vi "Debug Transceiver.vi"(11 "UDPlog Transceiver in":refnum<class "UDPlog Transceiver.lvclass">) -> (3 "UDPlog Transceiver out":refnum<class "UDPlog Transceiver.lvclass">)   [LabVIEW 2023, in "UDPlog.lvlib" / "UDPlog Transceiver.lvclass"]
uses:
  UDPlog Transceiver.lvclass
  UDPlog Transceiver.lvclass/UDPlog Transceiver.ctl
  <vilib>/Utility/SystemLogging/NI_SystemLogging.lvlib
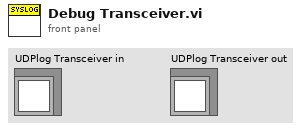
[diagram p1: front panel]
types:
  T1 = typedef "UDPlog.lvlib/UDPlog Transceiver.lvclass/Trasfer Group Parameters.ctl" = cluster{"transfers":T2[], "max size":i32, "timeout":i32}
  T2 = typedef "UDPlog.lvlib/UDPlog Transceiver.lvclass/Transfer Parameters.ctl" = cluster{"group offset":u64, "size":u64, "address":u32, "port":u16}
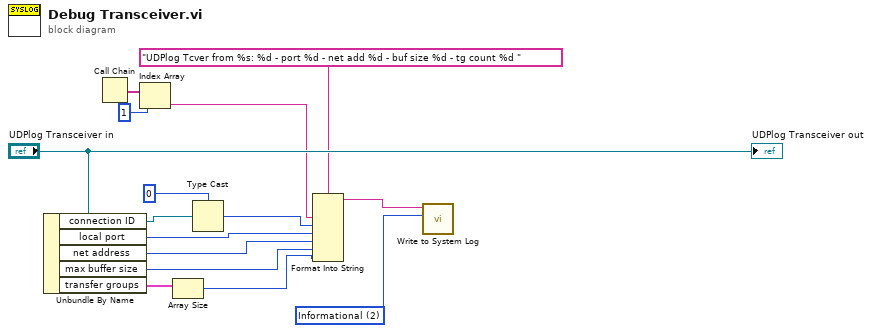
[diagram p0: block diagram]
diagram:
  w4 = 2 items=["Error", "Warning", "Informational"] ("severity")
  n1 = Unbundle By Name("UDPlog Transceiver in") -> ("connection ID"=w12:refnum<k16>, "local port"=w10:u16, "net address"=w9:u32, "max buffer size"=w8:u64, "transfer groups"=w7:T1[])
  n2 = Call Chain() -> (call chain=w3:string[])
  n3 = Index Array(array=w3, index=1) -> (element=w1:string)
  n4 = Array Size(array=w7) -> (size(s)=w6:i32)
  n5 = Type Cast(type=u64 0 ("unsigned 64bit integer"), x=w12) -> (*(type *) &x=w11:u64)
  n6 = Format Into String(format string="UDPlog Tcver from %s: %d - port %d - net add %d - buf size %d - tg count %d ", w1, w11, w10, w9, w8, w6) -> (resulting string=w5:string)  [unwired: 2 in, 1 out]
  n7 = call <vilib>:"Write to System Log.vi"("severity"=w4, "message"=w5) -> ()  [unwired: 9 in, 1 out]
  "UDPlog Transceiver out" <- "UDPlog Transceiver in"
